vi "fftw_malloc_cplx_double.vi"(8 "error in (no error)":errorcluster, 11 "cplx double count":u32=256) -> (0 "error out":errorcluster, 3 "*data":u64)   [LabVIEW 2020, in "FFTWDLL.lvlib"]
doc: "Allocate FFTW memory aligned for SIMD in complex double."
uses:
  FFTWDLL.lvlib
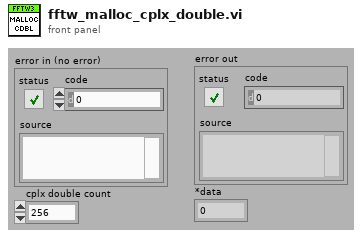
[diagram p1: front panel]
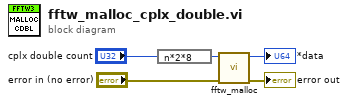
[diagram p0: block diagram]
diagram:
  n1 = expression code="n*2*8"("cplx double count") -> (w4:u32)
  n2 = call "fftw_malloc.vi"("error in (no error)"="error in (no error)", "bytes count"=w4) -> ("error out"=→"error out":errorcluster, "*data"=→"*data":u64)  [unwired: 8 in]
